vi "Export SQL.vi"(8 "error in (no error)":errorcluster, 10 "Export Data":T1, 11 "Import Export SQL in":refnum<class "Import Export SQL.lvclass">) -> (0 "error out":errorcluster, 3 "Import Export SQL out":refnum<class "Import Export SQL.lvclass">)   [LabVIEW 2023, in "Data Analysis.lvlib" / "Import Export SQL.lvlib" / "Import Export SQL.lvclass"]
uses:
  Import Export SQL.lvclass
  <vilib>/Utility/sysdir.llb/System Directory Type.ctl
  Import Export SQL.lvclass/Import Export SQL.ctl
  7eab2486-92b1-4603-aabd-00f400fbdcdf.vi
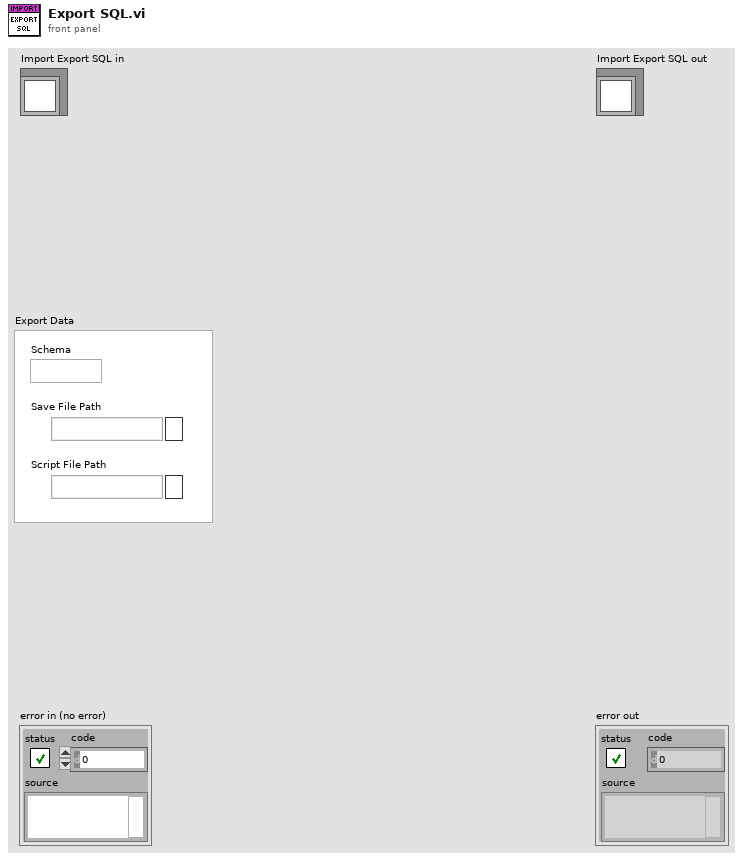
[diagram p1: front panel]
types:
  T1 = cluster{"Schema":string, "Save File Path":path, "Script File Path":path}
  T2 = typedef "System Directory Type.ctl" = i32
  T3 = enum16{"open", "replace", "create", "open or create", "replace or create", "replace or create with confirmation"}
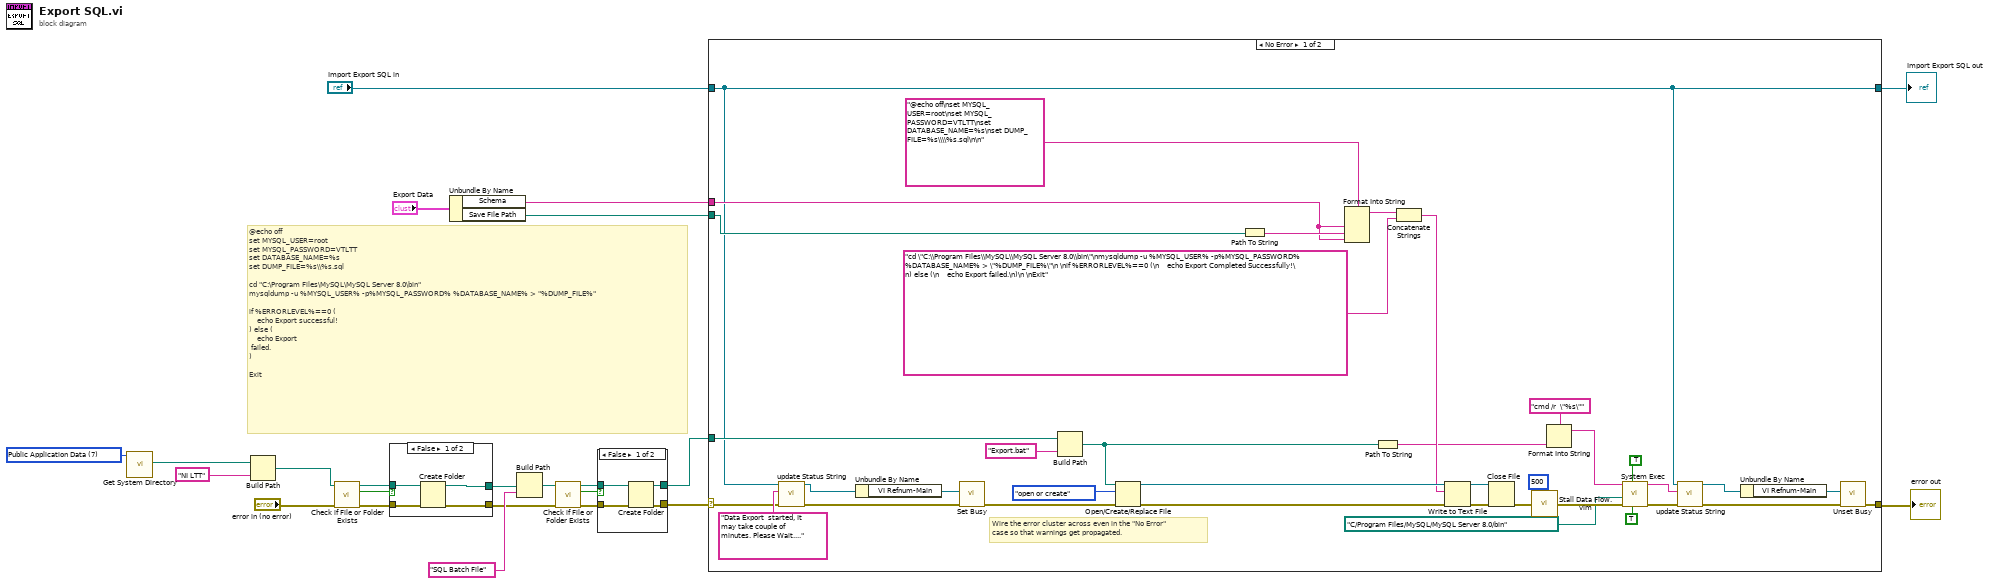
[diagram p0: block diagram]
diagram:
  w10 = T2 7 items=["User Home"=0, "User Desktop"=1, "User Documents"=2, "User Application Data"=3, "User Preferences"=4, "User Temporary"=5, "Public Documents"=6, "Public Application Data"=7, "Public Preferences"=8, "Public Cache"=13, "System Core Libraries"=9, "System Installed Libraries"=10, "Application Files"=11, "Boot Volume Root"=12] ("system directory type")
  # "@echo off\nset MYSQL_USER=root\nset MYSQL_PASSWORD=VTLTT\nset DATABASE_NAME=%s\nset DUMP_FILE=%s\\\\%s.sql\n\ncd \"C:\\Program Files\\MySQL\\MySQL Server 8.0\\bin\"\nmysqldump -u %MYSQL_USER% -p%MYSQL_PASSWORD% %DATABASE_NAME% > \"%DUMP_FILE%\"\n \nif %ERRORLEVEL%==0 (\n    echo Export successful!\n) else (\n    echo Export\n failed.\n)\n \nExit"
  n1 = call <vilib>:"Get System Directory.vi"("system directory type"=w10) -> ("system directory"=w11:path)  [unwired: 10 in]
  n2 = Build Path(base path=w11, name or relative path="NI LTT") -> (appended path=w6:path)
  n3 = call <vilib>:"Check if File or Folder Exists.vi"("error in (no error)"="error in (no error)", "path"=w6) -> ("error out"=w7:errorcluster, "file or folder exists?"=w8:bool, "dup path"=w9:path)  [unwired: 7 in]
  n4 = case shown="False" w8 {
    tunnel: w7 -> [w27 w29]
    tunnel: [w26 w29] -> w4
    tunnel: w9 -> [w25 w28]
    tunnel: [w24 w28] -> w5
    frame False {
      n5 = Create Folder(path (use dialog)=w25, error in=w27) -> (created path=w24:path, error out=w26:errorcluster)  [unwired: 1 in, 1 out]
    }
    frame True {
    }
  }
  n6 = Unbundle By Name("Export Data") -> ("Schema"=w19:string, "Save File Path"=w18:path)
  n7 = Build Path(base path=w5, name or relative path="SQL Batch File") -> (appended path=w15:path)
  n8 = call <vilib>:"Check if File or Folder Exists.vi"("error in (no error)"=w4, "path"=w15) -> ("error out"=w16:errorcluster, "file or folder exists?"=w14:bool, "dup path"=w13:path)  [unwired: 7 in]
  n9 = case shown="False" w14 {
    tunnel: w16 -> [w33 w35]
    tunnel: [w32 w35] -> w1
    tunnel: w13 -> [w31 w34]
    tunnel: [w30 w34] -> w3
    frame False {
      n10 = Create Folder(path (use dialog)=w31, error in=w33) -> (created path=w30:path, error out=w32:errorcluster)  [unwired: 1 in, 1 out]
    }
    frame True {
    }
  }
  n11 = case shown="No Error" w1 {
    selector: w1 -> [w42 w74]
    tunnel: [w50 w74] -> w23
    tunnel: [w38 w73] -> w21
    tunnel: "Import Export SQL in" -> [w38 w73]
    tunnel: w3 -> [w59 _]
    tunnel: w19 -> [w48 _]
    tunnel: w18 -> [w58 _]
    frame No Error {
      # "Wire the error cluster across even in the \"No Error\"\ncase so that warnings get propagated."
      n12 = call "update Status String.vi"("error in (no error)"=w42, "Data to Append"="Data Export  started, It may take couple of  minutes. Please Wait....", "Import Export SQL in"=w38) -> ("error out"=w41:errorcluster, "Import Export SQL out"=w44:refnum<class "Import Export SQL.lvclass">)  [unwired: 7 in]
      n13 = Unbundle By Name(w44) -> ("VI Refnum-Main"=w53:refnum<vi>)
      n14 = call <vilib>:"Set Busy.vi"("error in (no error)"=w41, "VI reference (current VI)"=w53) -> ("error out"=w52:errorcluster)  [unwired: 8 in, 1 out]
      n15 = Build Path(base path=w59, name or relative path="Export.bat") -> (appended path=w55:path)
      n16 = Open/Create/Replace File(file path (use dialog)=w55, error in=w52, operation (0:open)=T3."open or create") -> (refnum out=w72:refnum<file>, error out=w71:errorcluster)  [unwired: 3 in, 1 out]
      n17 = Path To String(path=w58) -> (string=w65:string)
      n18 = Format Into String(format string="@echo off\nset MYSQL_USER=root\nset MYSQL_PASSWORD=VTLTT\nset DATABASE_NAME=%s\nset DUMP_FILE=%s\\\\%s.sql\n\n", w48, w65, w48) -> (resulting string=w68:string)  [unwired: 2 in, 1 out]
      n19 = Path To String(path=w55) -> (string=w54:string)
      n20 = Concatenate Strings(w68, "cd \"C:\\Program Files\\MySQL\\MySQL Server 8.0\\bin\"\nmysqldump -u %MYSQL_USER% -p%MYSQL_PASSWORD% %DATABASE_NAME% > \"%DUMP_FILE%\"\n \nif %ERRORLEVEL%==0 (\n    echo Export Completed Successfully!\n) else (\n    echo Export failed.\n)\n \nExit") -> (w67:string)
      n21 = Write to Text File(file (use dialog)=w72, text=w67, error in=w71) -> (refnum out=w69:refnum<file>, error out=w70:errorcluster)  [unwired: 1 in, 1 out]
      n22 = Close File(refnum=w69, error in=w70) -> (error out=w64:errorcluster)  [unwired: 1 out]
      n23 = call "Stall Data Flow.vim"("value in"=w64, "milliseconds to wait"=u32 500) -> ("value out"=w62:errorcluster)  [unwired: 1 out]
      n24 = Format Into String(format string="cmd /r  \"%s\"" ("command line"), w54) -> (resulting string=w57:string)  [unwired: 2 in, 1 out]
      n25 = call <vilib>:"System Exec.vi"("run minimized? (F)"=TRUE, "wait until completion? (T)"=TRUE, "error in (no error)"=w62, "working directory"=path "C:/Program Files/MySQL/MySQL Server 8.0/bin", "command line"=w57) -> ("error out"=w40:errorcluster, "standard output"=w36:string)  [unwired: 3 in, 2 out]
      n26 = call "update Status String.vi"("error in (no error)"=w40, "Data to Append"=w36, "Import Export SQL in"=w38) -> ("error out"=w39:errorcluster, "Import Export SQL out"=w37:refnum<class "Import Export SQL.lvclass">)  [unwired: 7 in]
      n27 = Unbundle By Name(w37) -> ("VI Refnum-Main"=w51:refnum<vi>)
      n28 = call <vilib>:"Unset Busy.vi"("error in (no error)"=w39, "VI reference (current VI)"=w51) -> ("error out"=w50:errorcluster)  [unwired: 9 in]
    }
    frame Error {
    }
  }
  "error out" <- w23
  "Import Export SQL out" <- w21
